vi "rotate(NORMALNOE ROTATE).vi"(5 "I2C Ref in":T1, 7 "On/Off\nRight/Left":bool, 8 "error in (no error)":errorcluster) -> (0 "error out":errorcluster, 2 "I2C Ref out":T1)   [LabVIEW 2017]
uses:
  <vilib>/myRIO/Instrument Drivers/Onboard IO/I2C/typedefs/I2C Reference.ctl
  <vilib>/myRIO/Common/Instrument Driver Framework/Utilities/typedefs/myRIO Generic Hardware Reference.ctl
  <vilib>/myRIO/Common/Instrument Driver Framework/Utilities/typedefs/Hardware Version Enum.ctl
  <vilib>/myRIO/Common/Instrument Driver Framework/Utilities/typedefs/myRIO v1.0 Reference.ctl
  <vilib>/myRIO/Common/Instrument Driver Framework/Utilities/typedefs/Generic FPGA Reference.ctl
  <vilib>/myRIO/Common/Instrument Driver Framework/myRIO v1.0/I2C/typedefs/I2C Channels Enum.ctl
  <vilib>/myRIO/Instrument Drivers/Onboard IO/I2C/typedefs/I2C Configuration.ctl
  <vilib>/myRIO/Instrument Drivers/Onboard IO/I2C/typedefs/I2C Transfer Rate.ctl
  <vilib>/myRIO/Common/Instrument Driver Framework/myRIO v1.0/Encoder/typedefs/Encoder Signal Mode.ctl
  <vilib>/myRIO/Instrument Drivers/Onboard IO/Encoder/typedefs/Encoder Reference.ctl
  <vilib>/myRIO/Common/Instrument Driver Framework/myRIO v1.0/Encoder/typedefs/Encoder Channels Enum.ctl
  <vilib>/myRIO/Common/Instrument Driver Framework/myRIO v1.0/Encoder/typedefs/Encoder Configuration v1.0.ctl
  <vilib>/userdefined/High Color/nirio_resource_hc.ctl
  <vilib>/myRIO/Common/Instrument Driver Framework/Utilities/vis/Is FPGA Ref Available.vi
  <vilib>/myRIO/Common/Instrument Driver Framework/myRIO v1.0/Encoder/vis/myRIO v1.1 Open Encoder.vi
  <vilib>/myRIO/Instrument Drivers/Onboard IO/Encoder/vis/Read.vi
  <vilib>/myRIO/Common/Instrument Driver Framework/Utilities/vis/Validate Channels.vi
  <vilib>/myRIO/Common/Instrument Driver Framework/myRIO v1.0/Encoder/vis/myRIO v1.0 Reserve Encoder.vi
  <vilib>/myRIO/Common/Instrument Driver Framework/myRIO v1.0/Encoder/vis/myRIO v1.0 Build MUX Configuration Encoder.vi
  <vilib>/myRIO/Common/Instrument Driver Framework/myRIO v1.0/Resource Manager/vis/myRIO v1.0 Reserve Channel List.vi
  <vilib>/myRIO/Common/Instrument Driver Framework/myRIO v1.0/Resource Manager/vis/myRIO v1.0 Create Configuration List.vi
  <vilib>/myRIO/Common/Instrument Driver Framework/myRIO v1.0/Resource Manager/vis/myRIO v1.0 Reserve Channel.vi
  <vilib>/myRIO/Common/Instrument Driver Framework/myRIO v1.0/Resource Manager/vis/myRIO v1.0 Unreserve Channel.vi
  <vilib>/myRIO/Common/Instrument Driver Framework/myRIO v1.0/Resource Manager/vis/myRIO v1.0 Build Mutex Name.vi
  <vilib>/Utility/VariantDataType/GetNumericInfo.vi
  <vilib>/Utility/error.llb/Error Cluster From Error Code.vi
  <vilib>/myRIO/Common/Instrument Driver Framework/myRIO v1.0/myRIO v1.1 Open.vi
  <vilib>/myRIO/Common/Instrument Driver Framework/Utilities/vis/IO Manager.vi
  <vilib>/myRIO/Common/Instrument Driver Framework/Utilities/vis/Configuration Manager.vi
  <vilib>/myRIO/Common/Instrument Driver Framework/myRIO v1.0/Resource Manager/vis/myRIO v1.0 Configure IO.vi
  <vilib>/myRIO/Common/Instrument Driver Framework/myRIO v1.0/myRIO v1.0 Close.vi
  <vilib>/myRIO/Common/Instrument Driver Framework/myRIO v1.0/Encoder/vis/myRIO v1.0 Configure Encoder.vi
  <vilib>/myRIO/Common/Instrument Driver Framework/myRIO v1.0/Encoder/vis/myRIO v1.0 Read Encoder.vi
  <vilib>/imath/engines/lvmath2/RunTimeEngine/Managers/WorkSpace/UID Generator.vi
  <vilib>/imath/engines/lvmath2/RunTimeEngine/RunTimeType/NIMS_RunTimeType_From StrictType (excl LVString).vi
  <instcachedir>/0/NIMS_RunTimeType_From StrictType (excl LVString)_1019F277F0A747EDBCA0F6C52CA54500.lvgen/NIMS_RunTimeType_From StrictType (excl LVString)_1019F277F0A747EDBCA0F6C52CA54500_000.vi
  <vilib>/imath/engines/lvmath2/RunTimeEngine/LocalVariableDefStatement/MC_LocalVariableDefStatement_Display.vi
  <vilib>/imath/engines/lvmath2/RunTimeEngine/Managers/SymbolTable/Clear UID.vi
  <vilib>/imath/engines/lvmath2/RunTimeEngine/NodeEndStatement/NIMS_NodeEndStatement_Output.vi
  <instcachedir>/0/NIMS_NodeEndStatement_Output_53EC0D466D134D7ABD903AC30B43404B.lvgen/NIMS_NodeEndStatement_Output_53EC0D466D134D7ABD903AC30B43404B_013.vi
  <vilib>/imath/engines/lvmath2/RunTimeEngine/ErrorHandling/NIMS_Finalize Error.vi
  <vilib>/myRIO/Common/Instrument Driver Framework/myRIO v1.0/DIO/vis/myRIO v1.0 Write DIO.vi
  <vilib>/myRIO/Express VI/Onboard IO/Encoder/Encoder Express VI.xnode
  <vilib>/myRIO/Instrument Drivers/Onboard IO/Encoder/vis/myRIO Encoder Open.xnode
  <vilib>/myRIO/Common/Instrument Driver Framework/myRIO v1.0/Encoder/typedefs/Encoder Count Direction Enum.ctl
  <vilib>/myRIO/Instrument Drivers/Onboard IO/Encoder/Encoder.lvlib
  <vilib>/imath/engines/lvmath2/RunTimeEngine/Managers/SymbolTable/NIMS_WorkSpace.lvlib
  <vilib>/myRIO/Instrument Drivers/Onboard IO/DIO/DIO.lvlib
  <vilib>/myRIO/Instrument Drivers/Onboard IO/I2C/I2C.lvlib
panel:
  out "angle Z(coerset)":ext
  out "main angle":ext
  out "angle Z":ext
  out "zMax right":ext
  out "zMin right":ext
  in  "Stop Motor(true block)":bool
  out "zMin left":ext
  out "zMax left":ext
  in  "Stop Motor(false block)":bool
  in  "Stop Button":bool
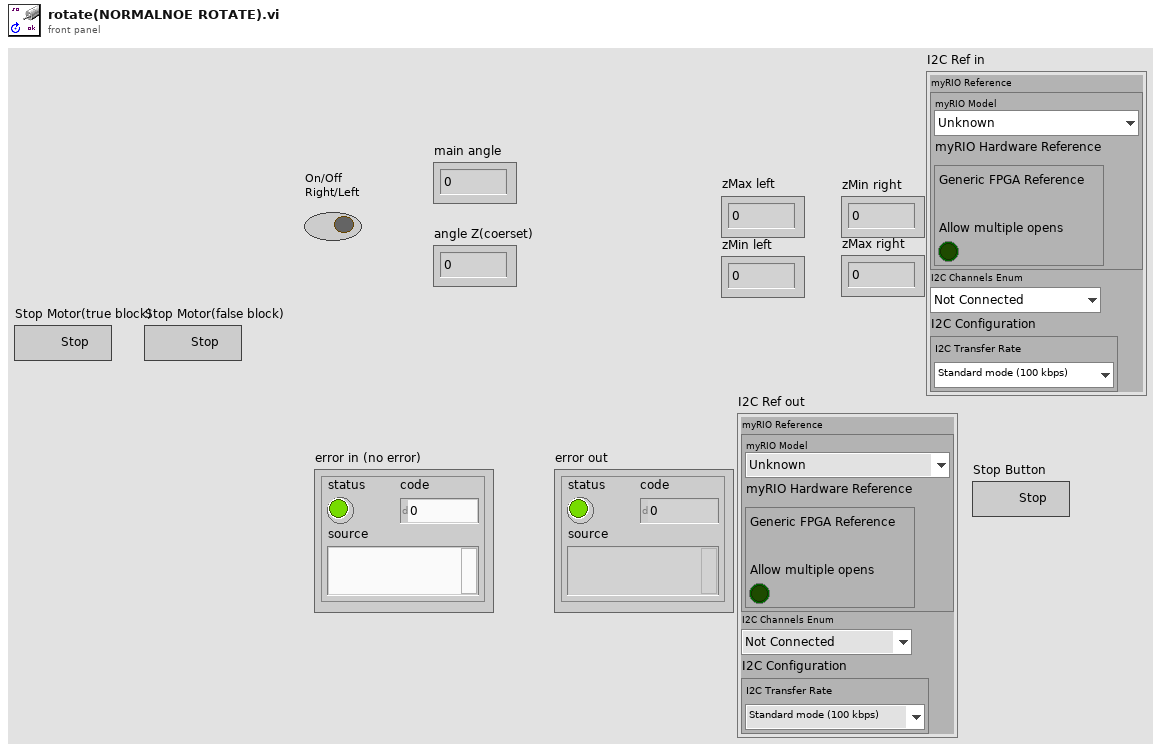
[diagram p1: front panel]
types:
  T1 = typedef "I2C.lvlib/I2C Reference.ctl" = cluster{"myRIO Reference":T2, "I2C Channels Enum":T6, "I2C Configuration":T7}
  T2 = typedef "myRIO Generic Hardware Reference.ctl" = cluster{"myRIO Model":T3, "myRIO Hardware Reference":T4}
  T3 = typedef "Hardware Version Enum.ctl" = enum16{"Unknown", "myRIO-1900", "myRIO-1950", "roboRIO", "NI ELVIS RIO CM"}
  T4 = typedef "myRIO v1.0 Reference.ctl" = cluster{"Generic FPGA Reference":T5, "Allow multiple opens":bool}
  T5 = typedef "Generic FPGA Reference.ctl" = refnum<k20>
  T6 = typedef "I2C Channels Enum.ctl" = enum16{"Not Connected", "A/I2C", "B/I2C", "I2C/I2C"}
  T7 = typedef "I2C.lvlib/I2C Configuration.ctl" = cluster{"I2C Transfer Rate":T8}
  T8 = typedef "I2C.lvlib/I2C Transfer Rate.ctl" = enum16{"Standard mode (100 kbps)", "Fast mode (400 kbps)"}
  T9 = typedef "DIO.lvlib/DIO Reference.ctl" = cluster{"myRIO Reference":T2, "DIO Channels List":T10}
  T10 = typedef "DIO Channels List.ctl" = T11[]
  T11 = typedef "DIO Channels Enum.ctl" = enum16{"Not Connected", "C/DIO0", "C/DIO1", "C/DIO2", "C/DIO3", "C/DIO4", "C/DIO5", "C/DIO6", "C/DIO7", "A/DIO0", "A/DIO1", "A/DIO2", "A/DIO3", "A/DIO4", "A/DIO5", "A/DIO6", "A/DIO7", "A/DIO8", "A/DIO9", "A/DIO10", "A/DIO11", "A/DIO12", "A/DIO13", "A/DIO14", "A/DIO15", "B/DIO0", "B/DIO1", "B/DIO2", "B/DIO3", "B/DIO4", "B/DIO5", "B/DIO6", "B/DIO7", "B/DIO8", "B/DIO9", "B/DIO10", "B/DIO11", "B/DIO12", "B/DIO13", "B/DIO14", "B/DIO15", "LED0", "LED1", "LED2", "LED3", "Button0", "DIO/DIO0", "DIO/DIO1", "DIO/DIO2", "DIO/DIO3", "DIO/DIO4", "DIO/DIO5", "DIO/DIO6", "DIO/DIO7", "DIO/DIO8", "DIO/DIO9", "SPI/CS0", "SPI/CS1", "SPI/CS2", "SPI/CS3", "LED RADIO (Green)", "LED RADIO (Red)", "LED COMM (Green)", "LED COMM (Red)", "LED MODE (Green)", "LED MODE (Red)"}
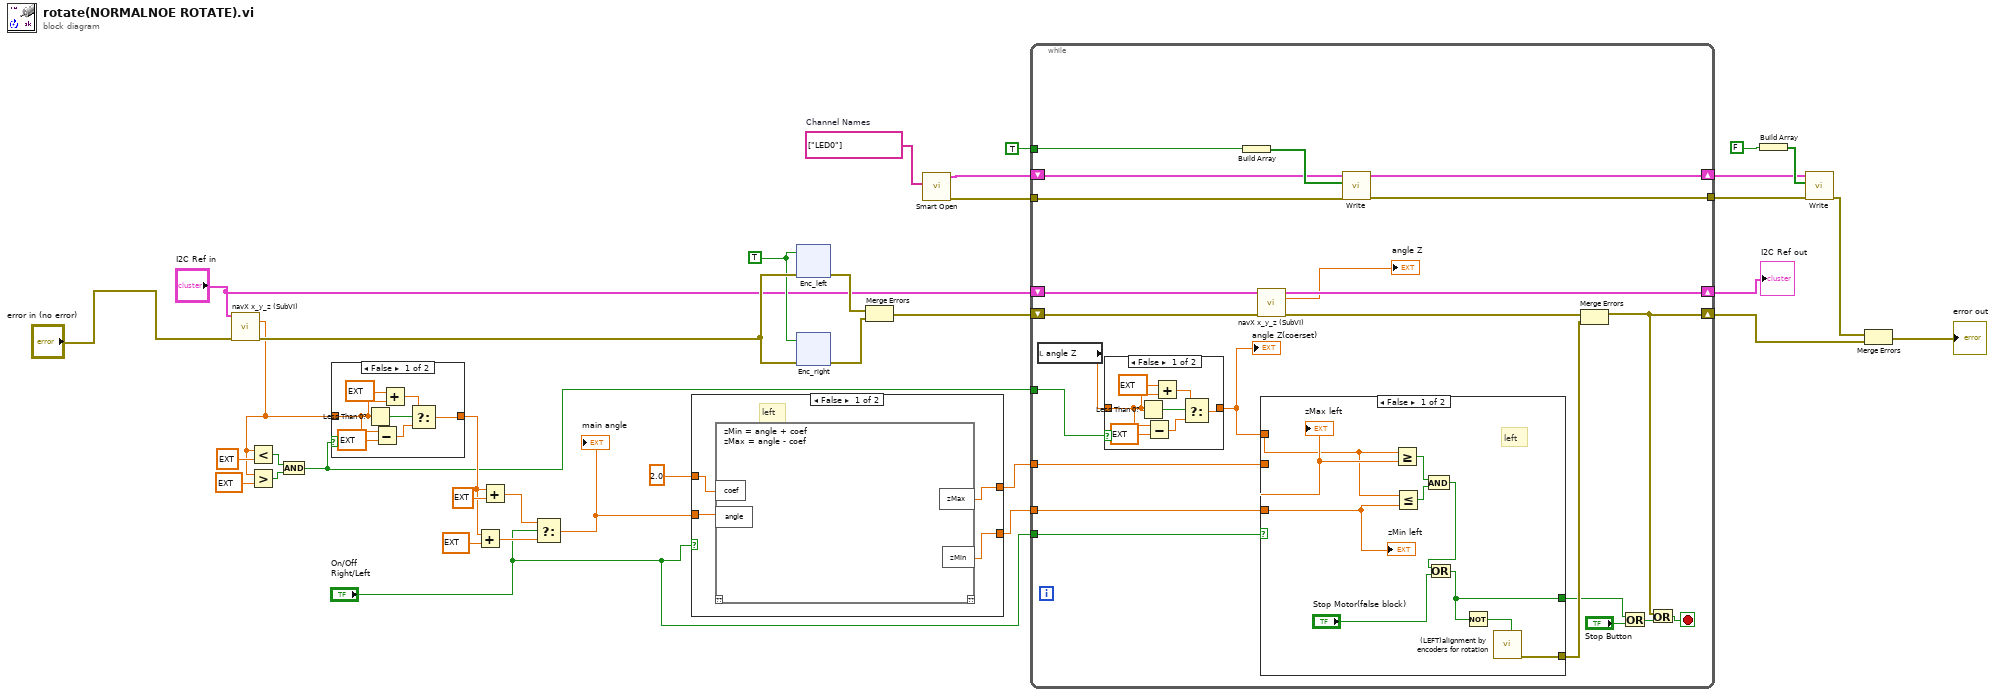
[diagram p0: block diagram]
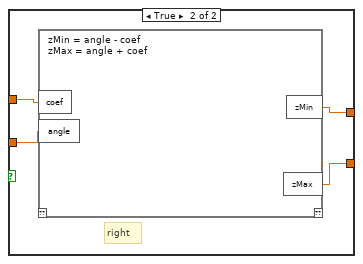
[diagram p3: hidden frame]
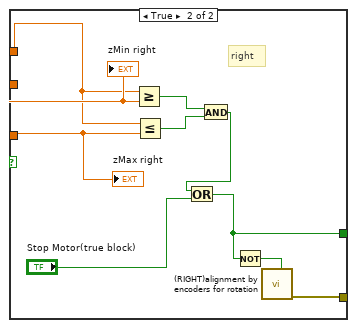
[diagram p5: hidden frame]
diagram:
  w13 = tag[] ["LED0"]  # Channel Names
  w26 = TRUE
  n1 = call "navX x_y_z (SubVI).vi"("I2C Ref Out in"="I2C Ref in", "error in (no error)"="error in (no error)") -> ("value Z"=w14:ext, "error out"=w27:errorcluster)  [unwired: 9 in, 3 out]
  n2 = Less?(x=w14, y=ext 90.0) -> (x < y?=w18:bool)
  n3 = Greater?(x=w14, y=ext -90.0) -> (0:w20:bool)
  n4 = And(x=w18, y=w20) -> (x .and. y?=w15:bool)
  n5 = case shown="False" w15 {
    tunnel: [w41 w43] -> w16
    tunnel: w14 -> [w36 w43]
    frame False {
      n6 = Less Than 0?(x=w36) -> (x < 0?=w42:bool)
      n7 = Subtract(x=w36, y=ext 180.0) -> (x-y=w38:ext)
      n8 = Add(x=ext 180.0, y=w36) -> (x+y=w40:ext)
      n9 = Select(t=w40, s=w42, f=w38) -> (s? t:f=w41:ext)
    }
    frame True {
    }
  }
  n10 = Add(x=w16, y=ext -90.0) -> (x+y=w31:ext)
  n11 = Add(x=w16, y=ext 90.0) -> (x+y=w30:ext)
  n12 = Select(t=w30, s="On/Off\nRight/Left", f=w31) -> (s? t:f=w17:ext)
  "main angle" <- w17
  n13 = case shown="False" "On/Off\nRight/Left" {
    tunnel: 2.0 ("coef") -> [w47 w106]
    tunnel: w17 -> [w46 w105]
    tunnel: [w44 w104] -> w24
    tunnel: [w45 w103] -> w23
    frame False {
      # "left"
      n14 = mathscript code="zMin = angle + coef\nzMax = angle - coef"("angle"=w46, "coef"=w47) -> ("zMin"=w45:ext, "zMax"=w44:ext)  [unwired: 1 in, 1 out]
    }
    frame True {
      # "right"
      n15 = mathscript code="zMin = angle - coef\nzMax = angle + coef"("angle"=w105, "coef"=w106) -> ("zMin"=w104:ext, "zMax"=w103:ext)  [unwired: 1 in, 1 out]
    }
  }
  n16 = xnode "Enc_left"("error in (no error)"=w27, "Reset Counter"=w26) -> ("error out"=w33:errorcluster)  [unwired: 3 out]
  n17 = xnode "Enc_right"("error in (no error)"=w27, "Reset Counter"=w26) -> ("error out"=w32:errorcluster)  [unwired: 3 out]
  n18 = Merge Errors(w33, w32) -> (w35:errorcluster)
  n19 = call <vilib>:"Smart Open.vi"("Channel Names"=w13) -> ("error out"=w8:errorcluster, "DIO Ref Out"=w6:T9)  [unwired: 9 in]
  n20 = while {
    shift-right: [w172] -> w1
    shift-left: w35 -> [w183]
    tunnel: "On/Off\nRight/Left" -> [w180]
    shift-right: [w179] -> w34
    shift-left: "I2C Ref in" -> [w184]
    tunnel: w24 -> [w176]
    tunnel: w23 -> [w175]
    tunnel: w15 -> [w169]
    tunnel: w8 -> [w164]
    tunnel: [w163] -> w7
    shift-right: [w166] -> w9
    shift-left: w6 -> [w165]
    tunnel: TRUE -> [w162]
    stop <- w173 stop-if-true
    n21 = local read "angle Z"() -> (w168:ext)
    n22 = case shown="False" w169 {
      tunnel: [w190 w192] -> w170
      tunnel: w168 -> [w185 w192]
      frame False {
        n23 = Less Than 0?(x=w185) -> (x < 0?=w191:bool)
        n24 = Subtract(x=w185, y=ext 180.0) -> (x-y=w187:ext)
        n25 = Add(x=ext 180.0, y=w185) -> (x+y=w189:ext)
        n26 = Select(t=w189, s=w191, f=w187) -> (s? t:f=w190:ext)
      }
      frame True {
      }
    }
    "angle Z(coerset)" <- w170
    n27 = Build Array(w162) -> (w167:bool[])
    n28 = call "navX x_y_z (SubVI).vi"("I2C Ref Out in"=w184, "error in (no error)"=w183) -> ("I2C Ref Out out"=w179:T1, "value Z"=→"angle Z":ext, "error out"=w181:errorcluster)  [unwired: 9 in, 2 out]
    n29 = case shown="False" w180 {
      tunnel: [w196 w207] -> w177
      tunnel: [w200 w206] -> w182
      tunnel: w176 -> [w194 w204]
      tunnel: w175 -> [w195 w205]
      tunnel: w170 -> [w193 w203]
      frame False {
        # "left"
        n30 = Greater Or Equal?(x=w193, y=w194) -> (x >= y?=w201:bool)
        n31 = Less Or Equal?(x=w193, y=w195) -> (x <= y?=w202:bool)
        n32 = And(x=w201, y=w202) -> (x .and. y?=w199:bool)
        n33 = Or(x=w199, y="Stop Motor(false block)") -> (x .or. y?=w196:bool)
        n34 = Not(x=w196) -> (.not. x?=w197:bool)
        n35 = call "(LEFT)alignment by encoders for rotation.vi"("On/Off"=w197) -> ("error out"=w200:errorcluster)  [unwired: 10 in]
        "zMin left" <- w195
        "zMax left" <- w194
      }
      frame True {
        # "right"
        n36 = Greater Or Equal?(x=w203, y=w204) -> (x >= y?=w212:bool)
        n37 = Less Or Equal?(x=w203, y=w205) -> (x <= y?=w211:bool)
        n38 = And(x=w212, y=w211) -> (x .and. y?=w210:bool)
        n39 = Or(x=w210, y="Stop Motor(true block)") -> (x .or. y?=w207:bool)
        n40 = Not(x=w207) -> (.not. x?=w208:bool)
        n41 = call "(RIGHT)alignment by encoders for rotation.vi"("On/Off"=w208) -> ("error out"=w206:errorcluster)  [unwired: 10 in]
        "zMax right" <- w205
        "zMin right" <- w204
      }
    }
    n42 = call <vilib>:"Write.vi"("error in (no error)"=w164, "Values"=w167, "DIO Ref In"=w165) -> ("error out"=w163:errorcluster, "DIO Ref Out"=w166:T9)  [unwired: 6 in]
    n43 = Merge Errors(w181, w182) -> (w172:errorcluster)
    n44 = Or(x=w177, y="Stop Button") -> (x .or. y?=w174:bool)
    n45 = Or(x=w172, y=w174) -> (x .or. y?=w173:bool)
  }
  "I2C Ref out" <- w34
  n46 = Build Array(FALSE) -> (w12:bool[])
  n47 = call <vilib>:"Write.vi"("error in (no error)"=w7, "Values"=w12, "DIO Ref In"=w9) -> ("error out"=w10:errorcluster)  [unwired: 6 in, 1 out]
  n48 = Merge Errors(w10, w1) -> (→"error out":errorcluster)
